vi "Read UUT Name.vi"(8 "error in":errorcluster, 11 "Base Software in":refnum<class "Main.lvclass">) -> (0 "error out":errorcluster, 2 "UUT_Name":string, 3 "Base Software out":refnum<class "Main.lvclass">)   [LabVIEW 2023, in "Main.lvlib" / "Main.lvclass"]
uses:
  Project/Main.lvclass
  Project/Main.lvclass/Main.ctl
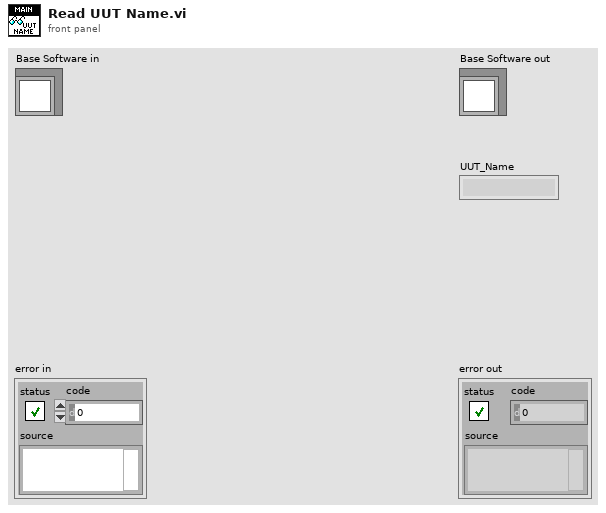
[diagram p1: front panel]
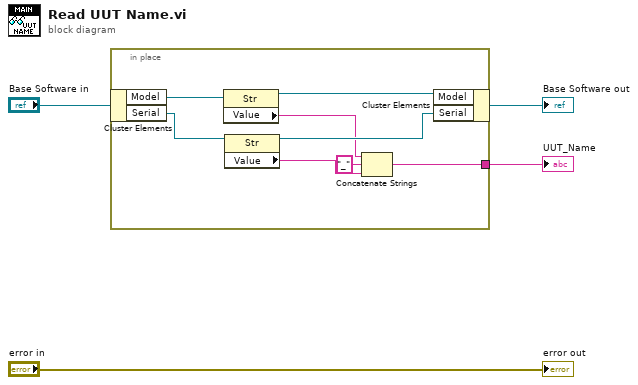
[diagram p0: block diagram]
diagram:
  n1 = in-place {
    in-place-border: [w5] -> w1
    n2 = in-place-cluster #1("Base Software in") -> ("Model"=w11:refnum<vi>, "Serial"=w12:refnum<vi>)
    n3 = property class="Str"(reference=w11) -> (reference out=w10:refnum<vi>, "Value"=w7:string)  [unwired: 1 in, 1 out]
    n4 = property class="Str"(reference=w12) -> (reference out=w9:refnum<vi>, "Value"=w6:string)  [unwired: 1 in, 1 out]
    n5 = Concatenate Strings(w7, "_" ("string"), w6) -> (w5:string)
    n6 = in-place-cluster #1("Model"=w10, "Serial"=w9) -> (→"Base Software out":refnum<class "Main.lvclass">)
  }
  "UUT_Name" <- w1
  "error out" <- "error in"
